vi "S8300E_PWOff_IP9258.vi"() -> ()   [LabVIEW 2011]
uses:
  Instance           6 33Saved   KT300WR2Base_ChkEUVersion .vi
panel:
  out "log":string
  out "Status狀況":string
  out "Begin Time":u32
  # "Power Off  IP9258"
  # "2014-12-1"
  # "需有 poweroff.bat\n本軟體程式是去呼叫WZS現有的IP9258程式"
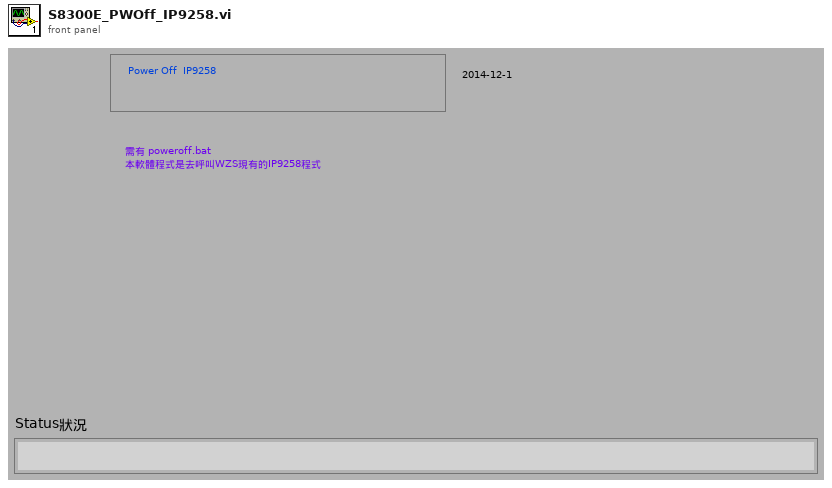
[diagram p1: front panel]
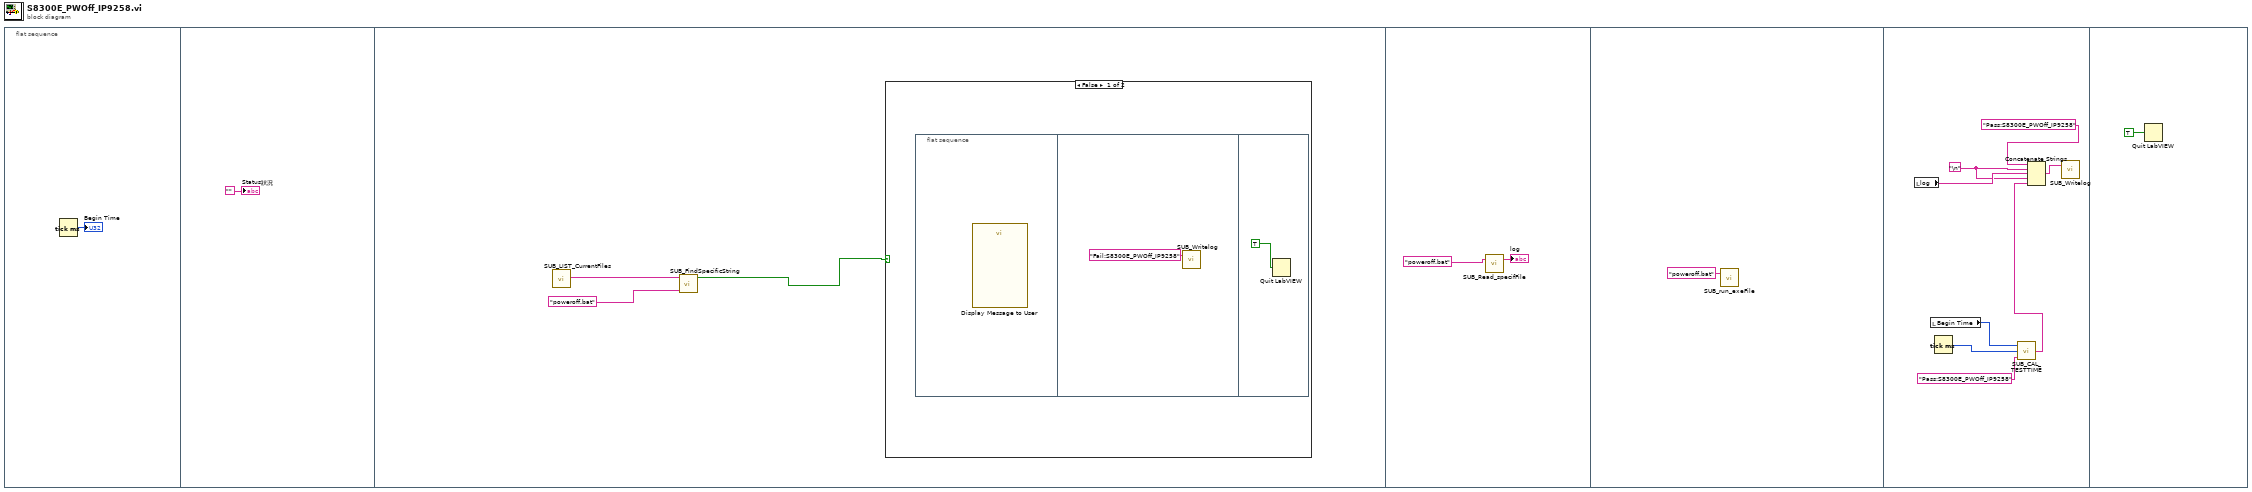
[diagram p0: block diagram]
diagram:
  n1 = flat-sequence {
    frame #0 {
      n2 = Tick Count (ms)() -> (millisecond timer value=→"Begin Time":u32)
    }
    frame #1 {
      "Status狀況" <- ""
    }
    frame #2 {
      n3 = call "SUB_LIST_CurrentFiles.vi"() -> ("To Upper Letters"=w5:string)  [unwired: 10 in, 1 out]
      n4 = call "SUB_FindSpecificString.vi"("Find this String"="poweroff.bat", "String data"=w5) -> ("Found"=w3:bool)  [unwired: 2 in, 1 out]
      n5 = case shown="False" w3 {
        frame False {
          n6 = flat-sequence {
            frame #0 {
              n7 = call "Display Message to User"() -> ()  [unwired: 10 in, 2 out]
            }
            frame #1 {
              n8 = call "SUB_Writelog.vi"("Pass/Fail"="Fail:S8300E_PWOff_IP9258") -> ()  [unwired: 2 in]
            }
            frame #2 {
              n9 = Quit LabVIEW(quit? (T)=TRUE) -> ()
            }
          }
        }
        frame True {
        }
      }
    }
    frame #3 {
      n10 = call "SUB_Read_specifFile.vi"("name or relative path"="poweroff.bat" ("exe filename")) -> ("text"=→"log":string)  [unwired: 1 in, 1 out]
    }
    frame #4 {
      n11 = call "SUB_run_exeFile.vi"("exe filename"="poweroff.bat") -> ()  [unwired: 2 in, 1 out]
    }
    frame #5 {
      w12 = "\n"
      n12 = local read "log"() -> (w13:string)
      n13 = local read "Begin Time"() -> (w16:u32)
      n14 = Tick Count (ms)() -> (millisecond timer value=w15:u32)
      n15 = call "SUB_CAL_TESTTIME.vi"("Test Item name"="Pass:S8300E_PWOff_IP9258" ("Pass/Fail"), "Stop tick time"=w15, "Start tick time"=w16) -> ("Test Time output"=w11:string)  [unwired: 2 in]
      n16 = Concatenate Strings("Pass:S8300E_PWOff_IP9258" ("Pass/Fail"), w12, w13, w12, w11) -> (w17:string)
      n17 = call "SUB_Writelog.vi"("Pass/Fail"=w17) -> ()  [unwired: 2 in]
    }
    frame #6 {
      n18 = Quit LabVIEW(quit? (T)=TRUE) -> ()
    }
  }
